vi "Identify.vi"(8 "error in (no error)":errorcluster, 11 "DCPower in":refnum<class "DCPower.lvclass">) -> (0 "error out":errorcluster, 2 "Plugin is Valid":bool, 3 "DCPower out":refnum<class "DCPower.lvclass">)   [LabVIEW 2018, in "DCPower.lvlib" / "DCPower.lvclass"]
uses:
  DCPower.lvclass
  C:/Sequence Automation/Plugins/Measurement Interface.lvlibp/Measurement Interface.lvclass
  Plugins/Measurement Interface.lvlibp/Private Methods/Measurement Definition Entry/Read Measurement Definition Entry.vi
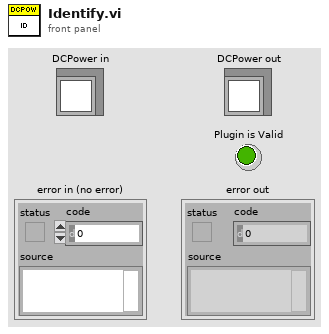
[diagram p1: front panel]
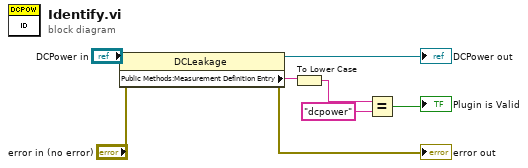
[diagram p0: block diagram]
diagram:
  n1 = property class="DCLeakage"(reference="DCPower in", error in="error in (no error)") -> (reference out=→"DCPower out":refnum<class "DCPower.lvclass">, error out=→"error out":errorcluster, "Public Methods:Measurement Definition Entry"=w4:string)
  n2 = To Lower Case(string=w4) -> (all lower case string=w2:string)
  n3 = Equal?(x=w2, y="dcpower") -> (x = y?=→"Plugin is Valid":bool)
